vi "SubVI_InitSide.vi"(0 "TalonCanID":u8, 1 "Invert output":bool=TRUE, 2 "sensor phase":bool=TRUE, 5 "Follow0CanID":u8=3, 7 "Follow1CanID":u8=2, 9 "Side":enum16{"Left", "Right"}(ring), 11 "error in (no error)":errorcluster) -> (4 "PhoenixMotorControlDevRef":T1, 15 "error out":errorcluster)   [LabVIEW 2017]
uses:
  <vilib>/Rock Robotics/WPI/MotorControl/WPI_MotorControlDeviceRef.ctl
  <vilib>/Rock Robotics/WPI/MotorControl/WPI_MotorControlType.ctl
  <vilib>/Rock Robotics/SystemInterfaces/DIO/FPGA_DIOPWMChannel.ctl
  <vilib>/Rock Robotics/WPI/PWM/WPI_PWMDeadband.ctl
  <vilib>/Rock Robotics/SystemInterfaces/DIO/FPGA_DIOChannel.ctl
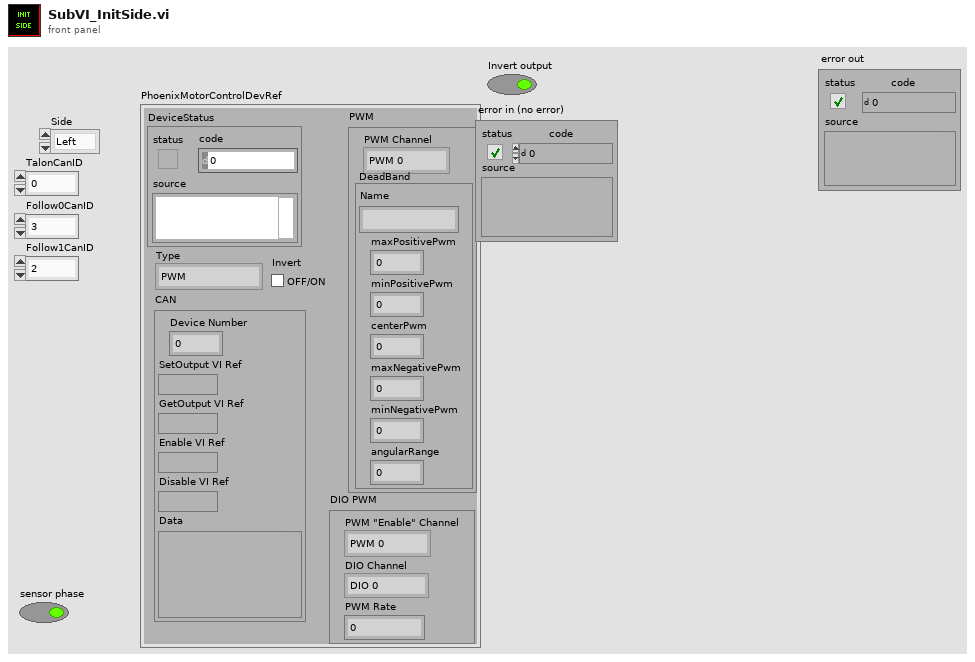
[diagram p1: front panel]
types:
  T1 = typedef "WPI_MotorControlDeviceRef.ctl" = cluster{"DeviceStatus":errorcluster, "Type":T2, "PWM":cluster{"PWM Channel":T3, "DeadBand":T4}, "CAN":cluster{"Device Number":u8, "SetOutput VI Ref":variant, "GetOutput VI Ref":variant, "Enable VI Ref":variant, "Disable VI Ref":variant, "Data":variant}, "Invert":bool, "DIO PWM":cluster{"PWM \"Enable\" Channel":T3, "DIOChannel":T5, "PWM Rate":dbl}}
  T2 = typedef "WPI_MotorControlType.ctl" = enum16{"PWM", "CAN", "DIO PWM"}
  T3 = typedef "FPGA_DIOPWMChannel.ctl" = enum8{"PWM 0", "PWM 1", "PWM 2", "PWM 3", "PWM 4", "PWM 5", "PWM 6", "PWM 7", "PWM 8", "PWM 9", "PWM MXP 0", "PWM MXP 1", "PWM MXP 2", "PWM MXP 3", "PWM MXP 4", "PWM MXP 5", "PWM MXP 6", "PWM MXP 7", "PWM MXP 8", "PWM MXP 9", "Invalid"}
  T4 = typedef "WPI_PWMDeadband.ctl" = cluster{"Name":string, "maxPositivePwm":i32, "minPositivePwm":i32, "centerPwm":i32, "maxNegativePwm":i32, "minNegativePwm":i32, "angularRange":u16}
  T5 = typedef "FPGA_DIOChannel.ctl" = enum8{"DIO 0", "DIO 1", "DIO 2", "DIO 3", "DIO 4", "DIO 5", "DIO 6", "DIO 7", "DIO 8", "DIO 9", "DIO MXP 0", "DIO MXP 1", "DIO MXP 2", "DIO MXP 3", "DIO MXP 4", "DIO MXP 5", "DIO MXP 6", "DIO MXP 7", "DIO MXP 8", "DIO MXP 9", "DIO MXP 10", "DIO MXP 11", "DIO MXP 12", "DIO MXP 13", "DIO MXP 14", "DIO MXP 15", "SPI Port CS1", "SPI Port CS2", "SPI Port CS3", "SPI Port MISO", "SPI Port MOSI", "Invalid"}
  T6 = enum16{"FollowerType_PercentOutput", "FollowerType_AuxOutput1"}
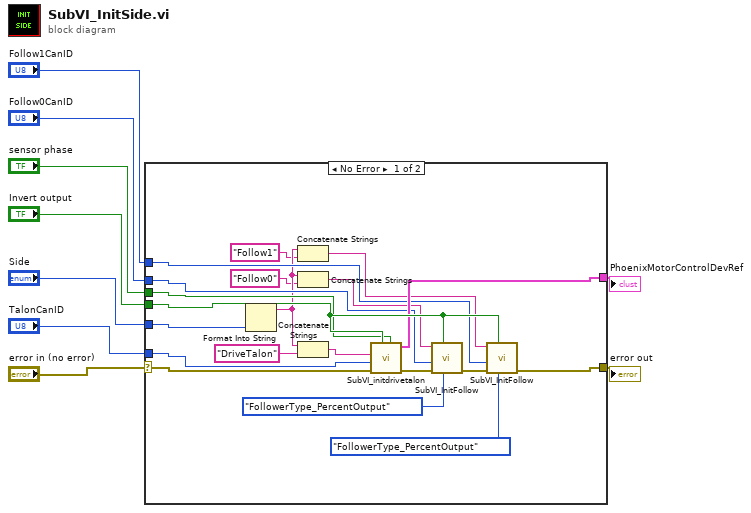
[diagram p0: block diagram]
diagram:
  n1 = case shown="No Error" "error in (no error)" {
    selector: "error in (no error)" -> [w27 w30]
    tunnel: "Invert output" -> [w29 _]
    tunnel: "sensor phase" -> [w28 _]
    tunnel: [w26 w30] -> w6
    tunnel: [w25 _] -> w5
    tunnel: "Side" -> [w24 _]
    tunnel: "TalonCanID" -> [w23 _]
    tunnel: "Follow0CanID" -> [w22 _]
    tunnel: "Follow1CanID" -> [w21 _]
    frame No Error {
      n2 = Format Into String(w24) -> (resulting string=w16:string)  [unwired: 3 in, 1 out]
      n3 = Concatenate Strings(w16, "Follow1" ("string")) -> (w13:string)
      n4 = Concatenate Strings(w16, "Follow0" ("string")) -> (w12:string)
      n5 = Concatenate Strings(w16, "DriveTalon" ("string")) -> (w17:string)
      n6 = call "SubVI_initdrivetalon.vi"("PhaseSensor"=w28, "Invert?"=w29, "error in (no error)"=w27, "Device Number"=w23, "refnum name"=w17) -> ("error out"=w20:errorcluster, "PhoenixMotorControlDevRef"=w25:T1)  [unwired: 5 in]
      n7 = call "SubVI_InitFollow.vi"("FollowerType"=T6."FollowerType_PercentOutput", "Invert?"=w29, "error in (no error)"=w20, "Can ID"=w22, "refnum name"=w12) -> ("error out"=w19:errorcluster)  [unwired: 6 in]
      n8 = call "SubVI_InitFollow.vi"("FollowerType"=T6."FollowerType_PercentOutput", "Invert?"=w29, "error in (no error)"=w19, "Can ID"=w21, "refnum name"=w13) -> ("error out"=w26:errorcluster)  [unwired: 6 in]
    }
    frame Error {
    }
  }
  "error out" <- w6
  "PhoenixMotorControlDevRef" <- w5
